vi "APS load parameter from flash.vi"(8 "error in (no error)":errorcluster caption="错误输入（无错误）", 11 "Board_ID":i32) -> (0 "error out":errorcluster caption="错误输出", 3 "function return":i32)   [LabVIEW 2012, in "APS168.lvlib"]
doc: "I32 FNTYPE APS_load_parameter_from_flash( I32 Board_ID );"
uses:
  APS168.lvlib
  APS168.dll
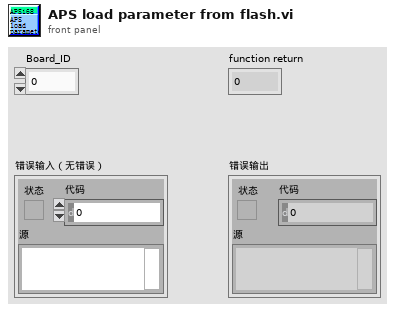
[diagram p1: front panel]
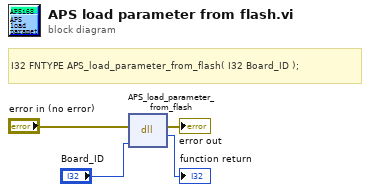
[diagram p0: block diagram]
diagram:
  # "I32 FNTYPE APS_load_parameter_from_flash( I32 Board_ID );"
  n1 = dll-call lib="PTH1,abs E\t冲压机运动204c\nAPS168.dll" fn="APS_load_parameter_from_flash"(error in="error in (no error)", "Board_ID"="Board_ID") -> (error out=→"error out":errorcluster, "返回类型"=→"function return":i32)  [unwired: 3 in, 1 out]
